vi "G#Debugger_FilterTrace.vi"(1 "TraceIn":string[](array[string]), 3 "FilterExpression":string) -> (15 "TraceOut":string[](array[string]))   [LabVIEW 2020, in "G#Debugger.lvlib"]
uses:
  G#Debugger.lvlib
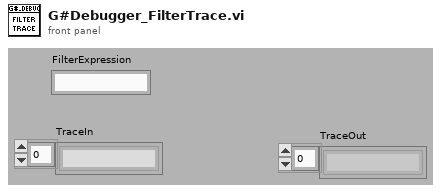
[diagram p1: front panel]
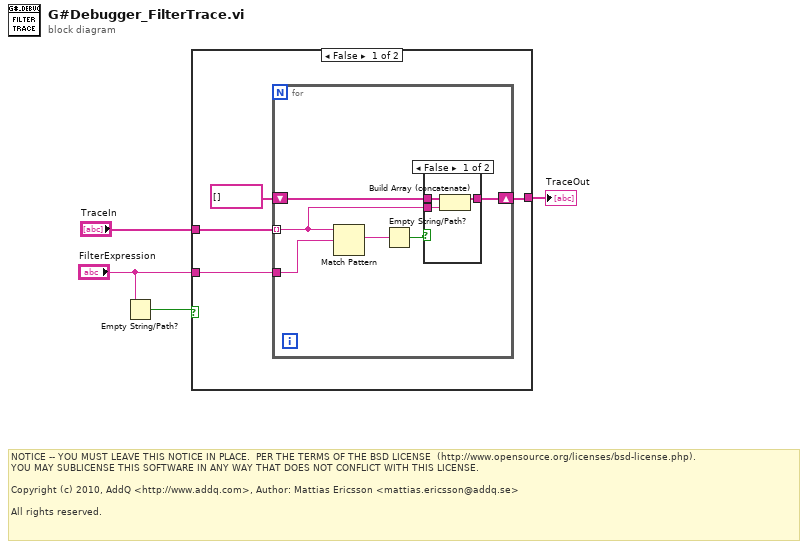
[diagram p0: block diagram]
diagram:
  # "NOTICE -- YOU MUST LEAVE THIS NOTICE IN PLACE.  PER THE TERMS OF THE BSD LICENSE  (http://www.opensource.org/licenses/bsd-license.php).\nYOU MAY SUBLICENSE THIS SOFTWARE IN ANY WAY THAT DOES NOT CONFLICT WITH THIS LICENSE.\n\nCopyright (c) 2010, AddQ <http://www.addq.com>, Author: Mattias Ericsson <mattias.ericsson@addq.se>\n\nAll rights reserved."
  n1 = Empty String/Path?(string/path="FilterExpression") -> (empty?=w3:bool)
  n2 = case shown="False" w3 {
    tunnel: "TraceIn" -> [w8 w19]
    tunnel: [w5 w19] -> w2
    tunnel: "FilterExpression" -> [w7 _]
    frame False {
      n3 = for {
        tunnel: w8 -> [w11] mode=indexing
        tunnel: w7 -> [w14]
        shift-right: [w9] -> w5
        shift-left: string[] [] ("TraceIn") -> [w12]
        n4 = Match Pattern(string=w11, regular expression=w14) -> (match substring=w13:string)  [unwired: 1 in, 3 out]
        n5 = Empty String/Path?(string/path=w13) -> (empty?=w10:bool)
        n6 = case shown="False" w10 {
          tunnel: w12 -> [w17 w18]
          tunnel: w11 -> [w16 _]
          tunnel: [w15 w18] -> w9
          frame False {
            n7 = Build Array (concatenate)(w17, w16) -> (w15:string[])
          }
          frame True {
          }
        }
      }
    }
    frame True {
    }
  }
  "TraceOut" <- w2
